vi "PathPlanner_Trajectory_CalculateRadius.vi"(9 "S2":T1={"AngularAcceleration"={"VALUE"=0.0, "COS"=1.0, "SIN"=0.0}, "PositionMeters"=0.0, "TrajectoryState"={"TimeSeconds"=0.0, "Velocity"=0.0, "Acceleration"=0.0, "POSE"={"TRANSLATION"={"X"=0.0, "Y"=0.0}, "ROTATION"={"VALUE"=0.0, "COS"=1.0, "SIN"=0.0}}, "Curvature"=0.0}, "AngularVelocity"={"VALUE"=0.0, "COS"=1.0, "SIN"=0.0}, "HolonomicRotation"={"VALUE"=0.0, "COS"=1.0, "SIN"=0.0}, "CurveRadius"=0.0, "DeltaPos"=0.0, "HolonomicAngular\nvelocity Deg/Sec"={"VALUE"=0.0, "COS"=1.0, "SIN"=0.0}} {"HolonomicAngular\nvelocity Deg/Sec"."SIN" format="%13.4f"; "HolonomicAngular\nvelocity Deg/Sec"."COS" format="%13.4f"; "HolonomicAngular\nvelocity Deg/Sec"."VALUE" format="%13.4f"; "HolonomicRotation"."SIN" format="%13.4f"; "HolonomicRotation"."COS" format="%13.4f"; "HolonomicRotation"."VALUE" format="%13.4f"; "AngularVelocity"."SIN" format="%13.4f"; "AngularVelocity"."COS" format="%13.4f"; "AngularVelocity"."VALUE" format="%13.4f"; "TrajectoryState"."POSE"."ROTATION"."SIN" format="%13.4f"; "TrajectoryState"."POSE"."ROTATION"."COS" format="%13.4f"; "TrajectoryState"."POSE"."ROTATION"."VALUE" format="%13.4f"; "TrajectoryState"."POSE"."TRANSLATION"."Y" format="%14.3f"; "TrajectoryState"."POSE"."TRANSLATION"."X" format="%14.3f"; "AngularAcceleration"."SIN" format="%13.4f"; "AngularAcceleration"."COS" format="%13.4f"; "AngularAcceleration"."VALUE" format="%13.4f"}, 10 "S1":T1={"AngularAcceleration"={"VALUE"=0.0, "COS"=1.0, "SIN"=0.0}, "PositionMeters"=0.0, "TrajectoryState"={"TimeSeconds"=0.0, "Velocity"=0.0, "Acceleration"=0.0, "POSE"={"TRANSLATION"={"X"=0.0, "Y"=0.0}, "ROTATION"={"VALUE"=0.0, "COS"=1.0, "SIN"=0.0}}, "Curvature"=0.0}, "AngularVelocity"={"VALUE"=0.0, "COS"=1.0, "SIN"=0.0}, "HolonomicRotation"={"VALUE"=0.0, "COS"=1.0, "SIN"=0.0}, "CurveRadius"=0.0, "DeltaPos"=0.0, "HolonomicAngular\nvelocity Deg/Sec"={"VALUE"=0.0, "COS"=1.0, "SIN"=0.0}} {"HolonomicAngular\nvelocity Deg/Sec"."SIN" format="%13.4f"; "HolonomicAngular\nvelocity Deg/Sec"."COS" format="%13.4f"; "HolonomicAngular\nvelocity Deg/Sec"."VALUE" format="%13.4f"; "HolonomicRotation"."SIN" format="%13.4f"; "HolonomicRotation"."COS" format="%13.4f"; "HolonomicRotation"."VALUE" format="%13.4f"; "AngularVelocity"."SIN" format="%13.4f"; "AngularVelocity"."COS" format="%13.4f"; "AngularVelocity"."VALUE" format="%13.4f"; "TrajectoryState"."POSE"."ROTATION"."SIN" format="%13.4f"; "TrajectoryState"."POSE"."ROTATION"."COS" format="%13.4f"; "TrajectoryState"."POSE"."ROTATION"."VALUE" format="%13.4f"; "TrajectoryState"."POSE"."TRANSLATION"."Y" format="%14.3f"; "TrajectoryState"."POSE"."TRANSLATION"."X" format="%14.3f"; "AngularAcceleration"."SIN" format="%13.4f"; "AngularAcceleration"."COS" format="%13.4f"; "AngularAcceleration"."VALUE" format="%13.4f"}, 11 "S0":T1={"AngularAcceleration"={"VALUE"=0.0, "COS"=1.0, "SIN"=0.0}, "PositionMeters"=0.0, "TrajectoryState"={"TimeSeconds"=0.0, "Velocity"=0.0, "Acceleration"=0.0, "POSE"={"TRANSLATION"={"X"=0.0, "Y"=0.0}, "ROTATION"={"VALUE"=0.0, "COS"=1.0, "SIN"=0.0}}, "Curvature"=0.0}, "AngularVelocity"={"VALUE"=0.0, "COS"=1.0, "SIN"=0.0}, "HolonomicRotation"={"VALUE"=0.0, "COS"=1.0, "SIN"=0.0}, "CurveRadius"=0.0, "DeltaPos"=0.0, "HolonomicAngular\nvelocity Deg/Sec"={"VALUE"=0.0, "COS"=1.0, "SIN"=0.0}} {"HolonomicAngular\nvelocity Deg/Sec"."SIN" format="%13.4f"; "HolonomicAngular\nvelocity Deg/Sec"."COS" format="%13.4f"; "HolonomicAngular\nvelocity Deg/Sec"."VALUE" format="%13.4f"; "HolonomicRotation"."SIN" format="%13.4f"; "HolonomicRotation"."COS" format="%13.4f"; "HolonomicRotation"."VALUE" format="%13.4f"; "AngularVelocity"."SIN" format="%13.4f"; "AngularVelocity"."COS" format="%13.4f"; "AngularVelocity"."VALUE" format="%13.4f"; "TrajectoryState"."POSE"."ROTATION"."SIN" format="%13.4f"; "TrajectoryState"."POSE"."ROTATION"."COS" format="%13.4f"; "TrajectoryState"."POSE"."ROTATION"."VALUE" format="%13.4f"; "TrajectoryState"."POSE"."TRANSLATION"."Y" format="%14.3f"; "TrajectoryState"."POSE"."TRANSLATION"."X" format="%14.3f"; "AngularAcceleration"."SIN" format="%13.4f"; "AngularAcceleration"."COS" format="%13.4f"; "AngularAcceleration"."VALUE" format="%13.4f"}) -> (3 "Radius":dbl)   [LabVIEW 2019, in "PathPlanner24.lvlib"]
uses:
  PathPlanner24.lvlib
  <vilib>/Rock Robotics/WPI/ThirdParty/JAS_Junk/TrajLib/Trajectory_Library.lvlib
  <vilib>/Rock Robotics/WPI/ThirdParty/JAS_Junk/TrajLib/TypeDef/ROTATION2D.ctl
  <vilib>/Rock Robotics/WPI/ThirdParty/JAS_Junk/TrajLib/TypeDef/TRANSLATION2D.ctl
  <vilib>/Rock Robotics/WPI/ThirdParty/JAS_Junk/TrajLib/TypeDef/POSE2D.ctl
  <vilib>/Rock Robotics/WPI/ThirdParty/JAS_Junk/TrajLib/TypeDef/TRAJ_STATE.ctl
  PathPlannerTrajectoryState.ctl
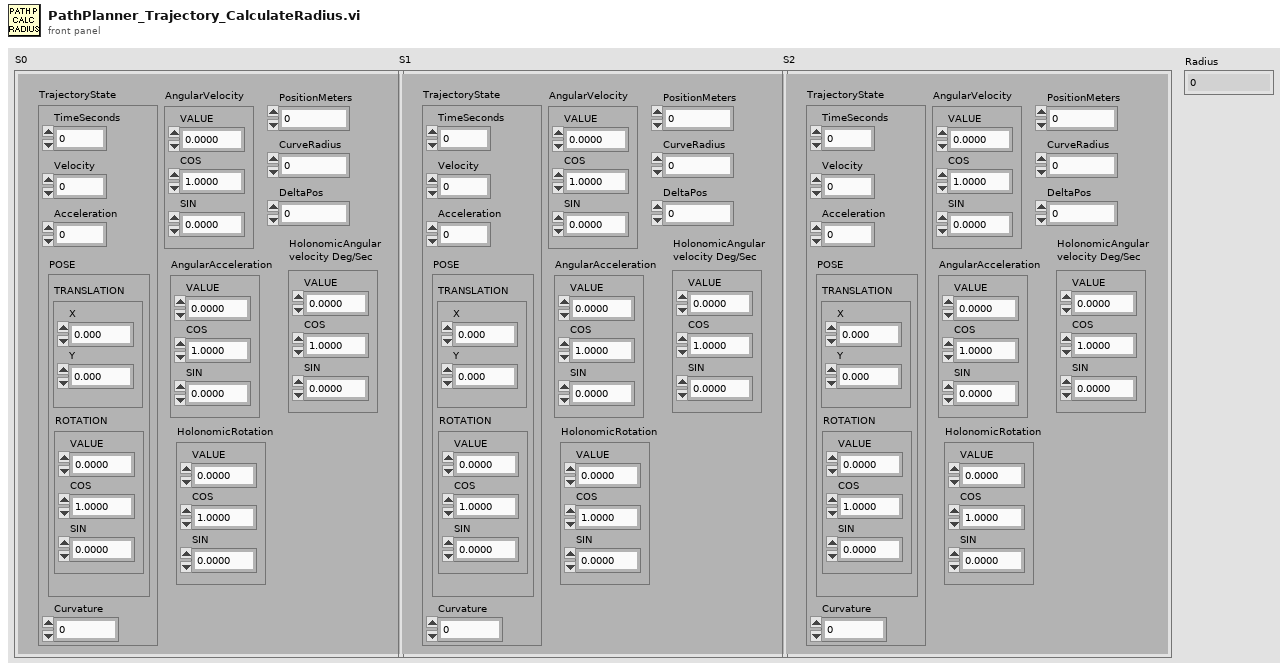
[diagram p1: front panel]
types:
  T1 = typedef "PathPlanner24.lvlib/PathPlannerTrajectoryState.ctl" = cluster{"AngularAcceleration":T2, "PositionMeters":dbl, "TrajectoryState":T3, "AngularVelocity":T2, "HolonomicRotation":T2, "CurveRadius":dbl, "DeltaPos":dbl, "HolonomicAngular\nvelocity Deg/Sec":T2}
  T2 = typedef "Trajectory_Library.lvlib/ROTATION2D.ctl" = cluster{"VALUE":dbl, "COS":dbl, "SIN":dbl}
  T3 = typedef "Trajectory_Library.lvlib/TRAJ_STATE.ctl" = cluster{"TimeSeconds":dbl, "Velocity":dbl, "Acceleration":dbl, "POSE":T4, "Curvature":dbl}
  T4 = typedef "Trajectory_Library.lvlib/POSE2D.ctl" = cluster{"TRANSLATION":T5, "ROTATION":T2}
  T5 = typedef "Trajectory_Library.lvlib/TRANSLATION2D.ctl" = cluster{"X":dbl, "Y":dbl}
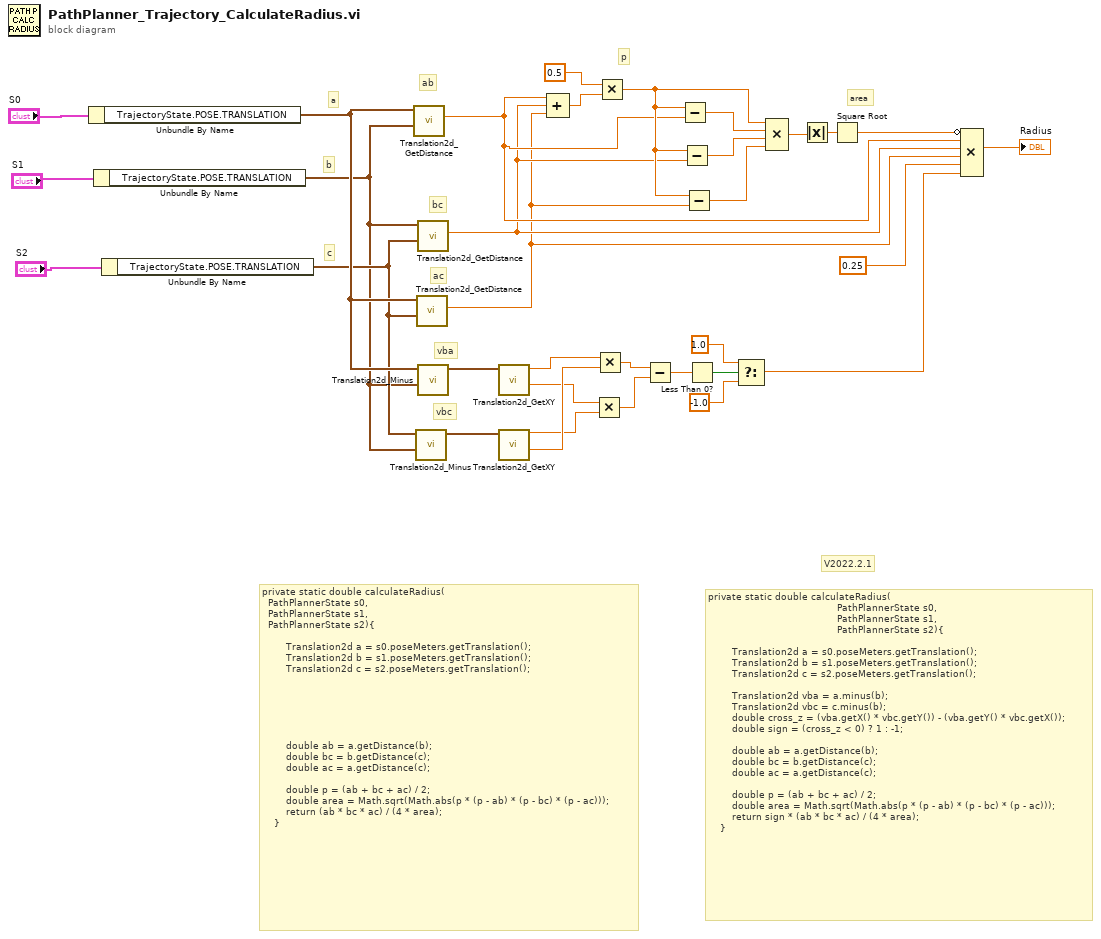
[diagram p0: block diagram]
diagram:
  # "vbc"
  # "vba"
  # "c"
  # "b"
  # "a"
  # "V2022.2.1"
  # "private static double calculateRadius(\n                                           PathPlannerState s0, \n                                           PathPlannerState s1, \n                                           PathPlannerState s2){\n\n        Translation2d a = s0.poseMeters.getTranslation();\n        Translation2d b = s1.poseMeters.getTranslation();\n        Translation2d c = s2.poseMeters.getTranslation();\n\n        Translation2d vba = a.minus(b);\n        Translation2d vbc = c.minus(b);\n        double cross_z = (vba.getX() * vbc.getY()) - (vba.getY() * vbc.getX());\n        double sign = (cross_z < 0) ? 1 : -1;\n\n        double ab = a.getDistance(b);\n        double bc = b.getDistance(c);\n        double ac = a.getDistance(c);\n\n        double p = (ab + bc + ac) / 2;\n        double area = Math.sqrt(Math.abs(p * (p - ab) * (p - bc) * (p - ac)));\n        return sign * (ab * bc * ac) / (4 * area);\n    }"
  # "private static double calculateRadius(\n\t\tPathPlannerState s0, \n\t\tPathPlannerState s1, \n\t\tPathPlannerState s2){\n\n        Translation2d a = s0.poseMeters.getTranslation();\n        Translation2d b = s1.poseMeters.getTranslation();\n        Translation2d c = s2.poseMeters.getTranslation();\n\n\n\n\n\n\n        double ab = a.getDistance(b);\n        double bc = b.getDistance(c);\n        double ac = a.getDistance(c);\n\n        double p = (ab + bc + ac) / 2;\n        double area = Math.sqrt(Math.abs(p * (p - ab) * (p - bc) * (p - ac)));\n        return (ab * bc * ac) / (4 * area);\n    }"
  # "area"
  # "p"
  # "ac"
  # "bc"
  # "ab"
  n1 = Unbundle By Name("S0") -> ("TrajectoryState.POSE.TRANSLATION"=w16:T5)
  n2 = Unbundle By Name("S1") -> ("TrajectoryState.POSE.TRANSLATION"=w14:T5)
  n3 = Unbundle By Name("S2") -> ("TrajectoryState.POSE.TRANSLATION"=w15:T5)
  n4 = call <vilib>:"Translation2d_GetDistance.vi"("other Translation"=w14, "In Translation"=w16) -> ("Distance"=w21:dbl)  [unwired: 9 in]
  n5 = call <vilib>:"Translation2d_Minus.vi"("other Translation"=w14, "In Translation"=w15) -> ("Out Translation"=w12:T5)  [unwired: 9 in]
  n6 = call <vilib>:"Translation2d_GetDistance.vi"("other Translation"=w15, "In Translation"=w16) -> ("Distance"=w19:dbl)  [unwired: 9 in]
  n7 = call <vilib>:"Translation2d_GetDistance.vi"("other Translation"=w15, "In Translation"=w14) -> ("Distance"=w20:dbl)  [unwired: 9 in]
  n8 = call <vilib>:"Translation2d_Minus.vi"("other Translation"=w14, "In Translation"=w16) -> ("Out Translation"=w13:T5)  [unwired: 9 in]
  n9 = call <vilib>:"Translation2d_GetXY.vi"("In Translation"=w13) -> ("Y"=w9:dbl, "X"=w11:dbl)  [unwired: 9 in]
  n10 = call <vilib>:"Translation2d_GetXY.vi"("In Translation"=w12) -> ("Y"=w10:dbl, "X"=w8:dbl)  [unwired: 9 in]
  n11 = Compound Arithmetic op=ADD(w21, w20, w19) -> (w30:dbl)
  n12 = Multiply(x=w9, y=w8) -> (x*y=w6:dbl)
  n13 = Multiply(x=w11, y=w10) -> (x*y=w7:dbl)
  n14 = Multiply(x=0.5, y=w30) -> (x*y=w28:dbl)
  n15 = Subtract(x=w7, y=w6) -> (x-y=w5:dbl)
  n16 = Subtract(x=w28, y=w21) -> (x-y=w27:dbl)
  n17 = Subtract(x=w28, y=w20) -> (x-y=w26:dbl)
  n18 = Subtract(x=w28, y=w19) -> (x-y=w25:dbl)
  n19 = Less Than 0?(x=w5) -> (x < 0?=w4:bool)
  n20 = Select(t=1.0, s=w4, f=-1.0) -> (s? t:f=w1:dbl)
  n21 = Compound Arithmetic op=MULTIPLY(w28, w27, w26, w25) -> (w24:dbl)
  n22 = Absolute Value(x=w24) -> (abs(x)=w23:dbl)
  n23 = Square Root(x=w23) -> (sqrt(x)=w22:dbl)
  n24 = Compound Arithmetic op=MULTIPLY(invert w22, w21, w20, w19, 0.25 ("value"), w1) -> (→"Radius":dbl)
